vi "Get Selected Edge Annotation Shown.vi"(8 "error in (no error)":errorcluster, 11 "FSM in":refnum<class "FSM.Graph.lvclass">) -> (0 "error out":errorcluster, 2 "shown":bool, 3 "FSM out":refnum<class "FSM.Graph.lvclass">)   [LabVIEW 2015, in "FSM.Graph.lvclass"]
uses:
  FSM.Graph.lvclass
  FSM.Graph.lvclass/FSM.Graph.ctl
  FSM.Edge/FSM.Edge.lvclass
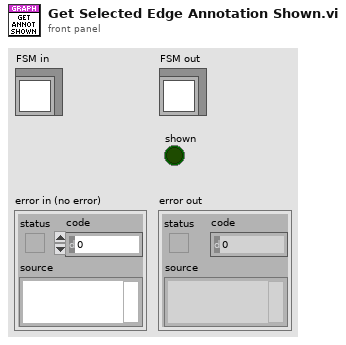
[diagram p1: front panel]
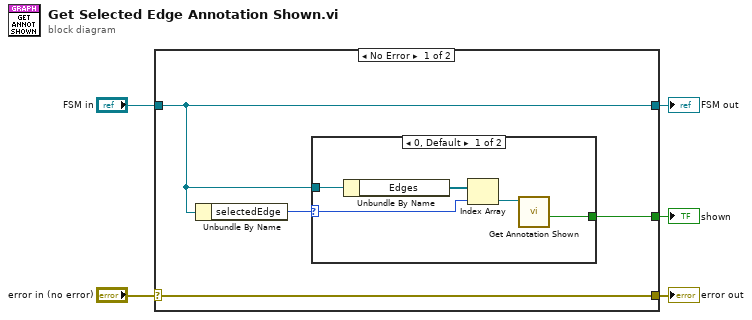
[diagram p0: block diagram]
diagram:
  n1 = case shown="No Error" "error in (no error)" {
    selector: "error in (no error)" -> [w9 w16]
    tunnel: [w9 w16] -> w4
    tunnel: [w7 w15] -> w2
    tunnel: "FSM in" -> [w7 w15]
    tunnel: [w6 _] -> w1
    frame No Error {
      n2 = Unbundle By Name(w7) -> ("selectedEdge"=w8:i32)
      n3 = case shown="0, Default" w8 {
        selector: w8 -> [w13 _]
        tunnel: w7 -> [w14 _]
        tunnel: [w10 _] -> w6
        frame 0, Default {
          n4 = Unbundle By Name(w14) -> ("Edges"=w12:refnum<class "FSM.Edge.lvclass">[])
          n5 = Index Array(array=w12, index=w13) -> (element=w11:refnum<class "FSM.Edge.lvclass">)
          n6 = call "Get Annotation Shown.vi"("FSM.Edge in"=w11) -> ("shown"=w10:bool)  [unwired: 8 in, 2 out]
        }
        frame -1 {
        }
      }
    }
    frame Error {
    }
  }
  "error out" <- w4
  "FSM out" <- w2
  "shown" <- w1
